vi "detach subscriber.vi"(8 "error in":errorcluster, 10 "stream publisher":refnum<class "data bus stream subscriber.lvclass">, 11 "stream publisher in":refnum<class "data bus stream publisher.lvclass">) -> (0 "error out":errorcluster, 3 "stream publisher out":refnum<class "data bus stream publisher.lvclass">)   [LabVIEW 2013, in "data bus stream publisher.lvclass"]
uses:
  data bus stream publisher.lvclass
  subscriber/data bus stream subscriber.lvclass
  data bus stream publisher.lvclass/data bus stream publisher.ctl
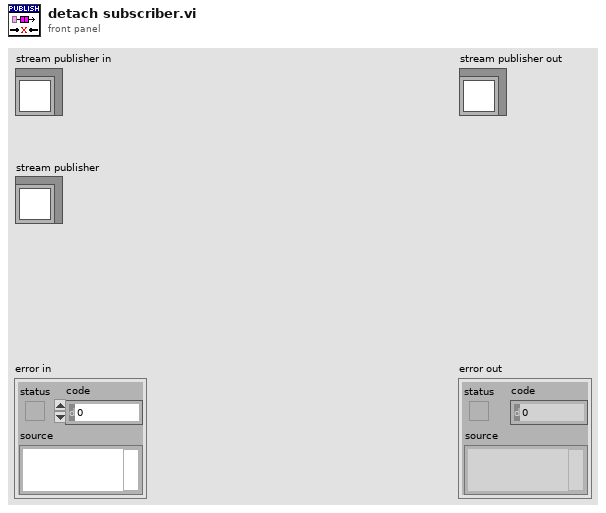
[diagram p1: front panel]
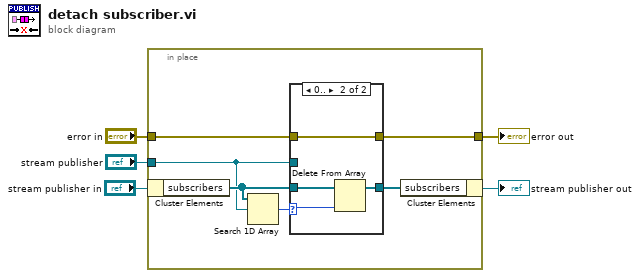
[diagram p0: block diagram]
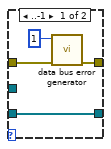
[diagram p2: hidden frame]
diagram:
  n1 = in-place {
    in-place-border: "stream publisher" -> [w6]
    in-place-border: "error in" -> [w10]
    in-place-border: [w9] -> w1
    n2 = in-place-cluster #1("stream publisher in") -> ("subscribers"=w7:refnum<class "data bus stream subscriber.lvclass">[])
    n3 = Search 1D Array(1D array=w7, element=w6) -> (index of element=w11:i32)  [unwired: 1 in]
    n4 = case shown="0.." w11 {
      selector: w11 -> [_ w17]
      tunnel: w10 -> [w15 w19]
      tunnel: [w14 w19] -> w9
      tunnel: [w12 w16] -> w8
      tunnel: w7 -> [w12 w18]
      tunnel: w6 -> [_ _]
      frame ..-1 {
        n5 = call "data bus error generator.vi"("error in"=w15, "error code (0)"=1) -> ("error out"=w14:errorcluster)  [unwired: 7 in]
      }
      frame 0.. {
        n6 = Delete From Array(array=w18, index=w17) -> (array with subset deleted=w16:refnum<class "data bus stream subscriber.lvclass">[])  [unwired: 1 in, 1 out]
      }
    }
    n7 = in-place-cluster #1("subscribers"=w8) -> (→"stream publisher out":refnum<class "data bus stream publisher.lvclass">)
  }
  "error out" <- w1
